vi "Main.vi"() -> ()   [LabVIEW 2020]
uses:
  Def/MHL_Data.ctl
  Def/Queue_Function Def.ctl
  Def/Queue_Method Def.ctl
  Def/Saving Type.ctl
  Def/Return(Watch Dog).ctl
  Def/Event Log.ctl
  Def/Error handler.ctl
  Objects/Saving Function/Saving OO/Save as csv/Save as csv.lvclass
  D:/Projects/practice/QMH+Producer_consumer/Multiple queues_PS/Objects/Saving Function/Saving OO/Saving OO.lvclass
  Def/Queue_Def.ctl
  <userlib>/_MGI/Timing/MGI Wait/MGI Wait (U32).vi
  Objects/Saving Function/Saving OO/Save as txt/Save as txt.lvclass
  Objects/Saving Function/Saving OO/Saving OO.lvclass
panel:
  in  "Connect/Reconnect":bool
  in  "Power":bool
  in  "Decrease Amplitude":bool
  in  "Add Amplitude":bool
  in  "Decrease Frequence":bool
  in  "Increase Frequence":bool
  out "Waveform":dynamicdata(graph)
  in  "MHL Data":T1={"Offset"=0.0, "Frequency"=10.1, "Amplitude"=1.0}
  out "Ver.#":string
  out "error out":errorcluster
  in  "error in (no error)":errorcluster
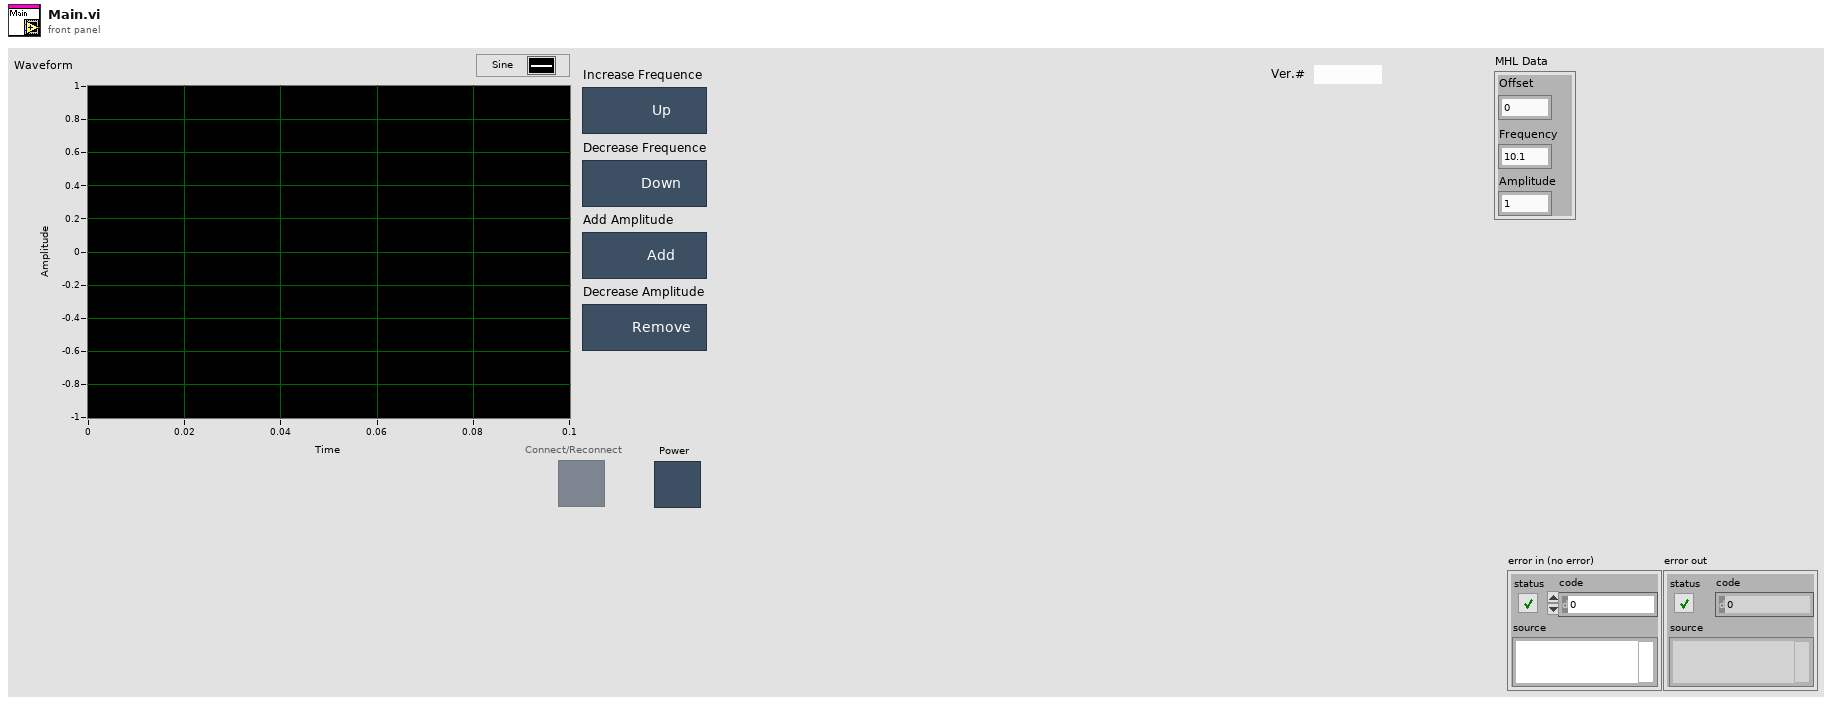
[diagram p1: front panel]
types:
  T1 = typedef "MHL_Data.ctl" = cluster{"Offset":dbl, "Frequency":dbl, "Amplitude":dbl}
  T2 = typedef "Error handler.ctl" = cluster{"code":i32, "source":string}
  T3 = typedef "Event Log.ctl" = cluster{"File paht":path}
  T4 = typedef "Queue_Method Def.ctl" = enum16{"Initialize", "Read", "Write", "Insert", "Get_Specific_Quene_Status", "Flush Speciffic Quene", "Release All Quenes"}
  T5 = typedef "Queue_Function Def.ctl" = enum16{"MHL", "Return(Watch dog)", "Event Log", "Error Log"}
  T6 = typedef "Return(Watch Dog).ctl" = cluster{string}
  T7 = typedef "Saving Type.ctl" = enum16{"Default", "txt", "csv"}
  T8 = typedef "Main_Data_Package.ctl" = cluster{"This Vi Ref Out":refnum<vi>, "Map Out":map{string, refnum<vi>}, "User Event Ref":refnum<user-event>, "User_Event Reg":refnum<event-registration>, "Event Log Path":path}
  T9 = enum8{"Enabled", "Disabled", "Disabled and Grayed Out"}
  T10 = typedef "Queue_Def.ctl" = cluster{"Message":string, "Data":variant}
  T11 = cluster{"Functions":T5, "Functions 2":T5, "Functions 3":T5, "Functions 4":T5}
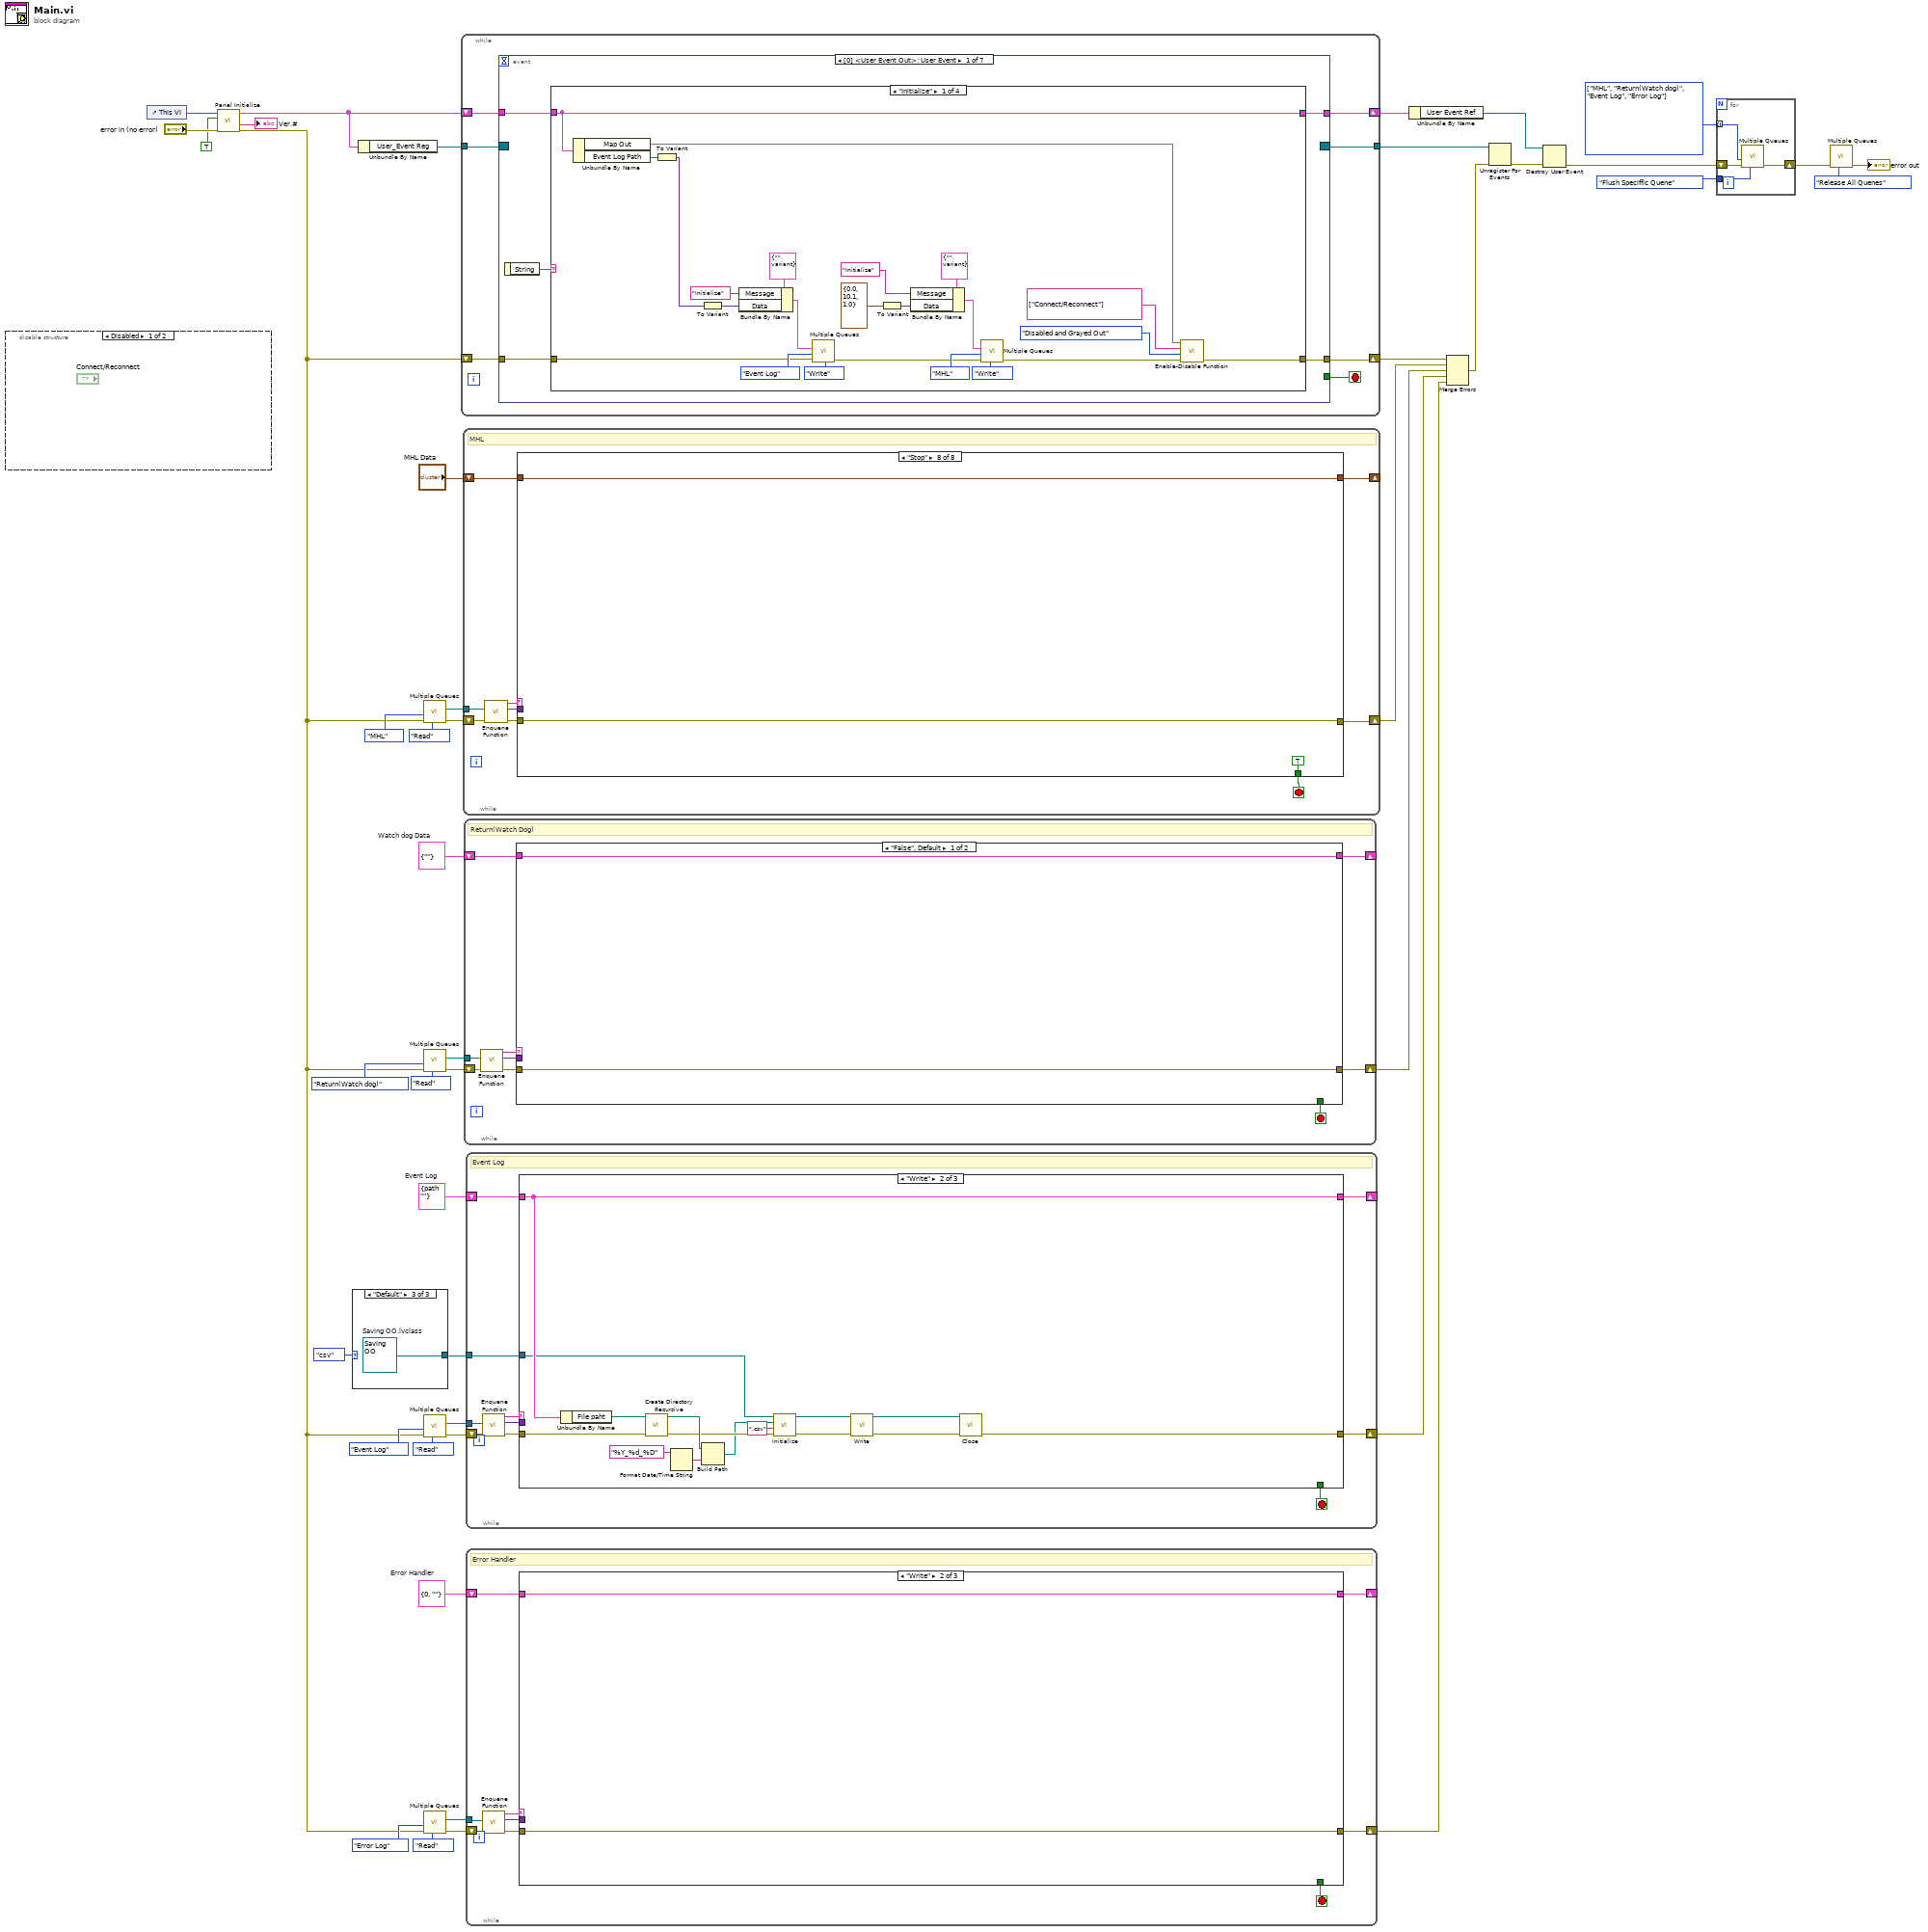
[diagram p0: block diagram]
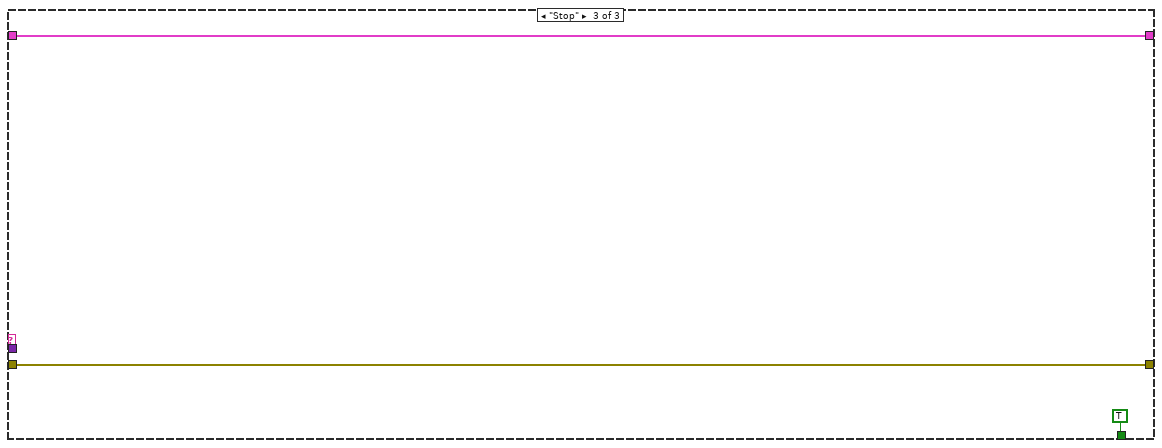
[diagram p3: hidden frame]
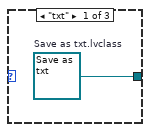
[diagram p5: hidden frame]
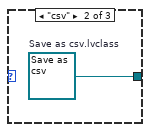
[diagram p6: hidden frame]
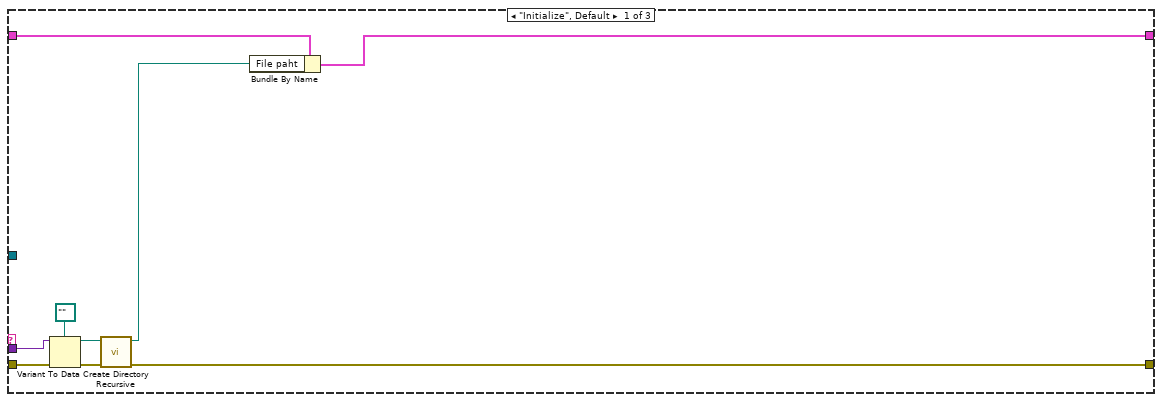
[diagram p7: hidden frame]
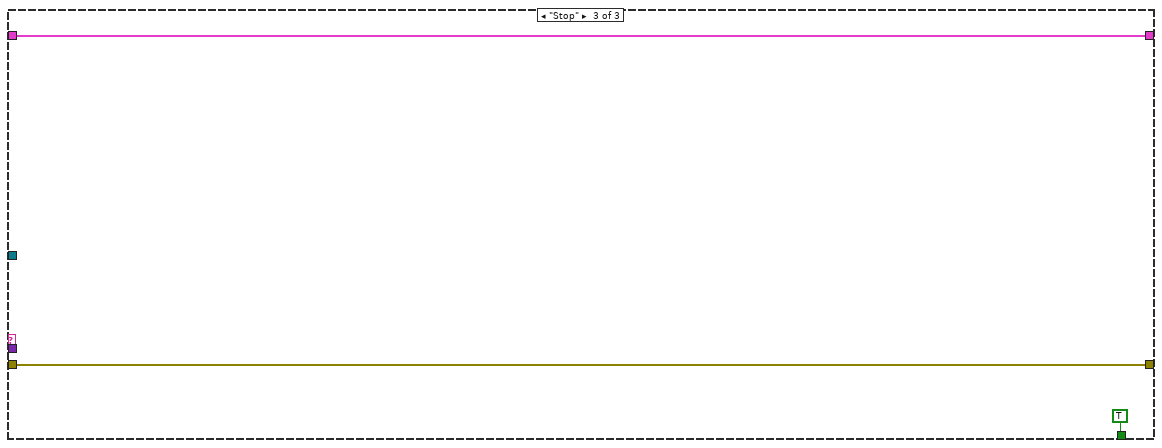
[diagram p8: hidden frame]
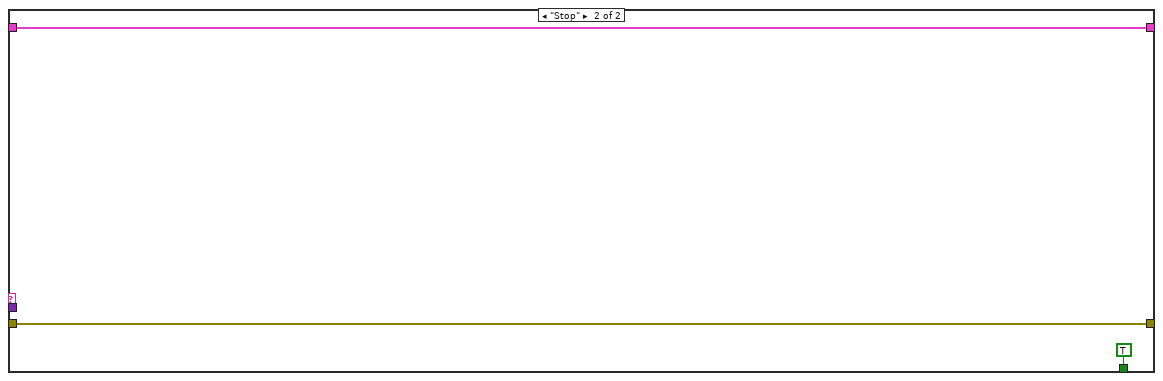
[diagram p9: hidden frame]
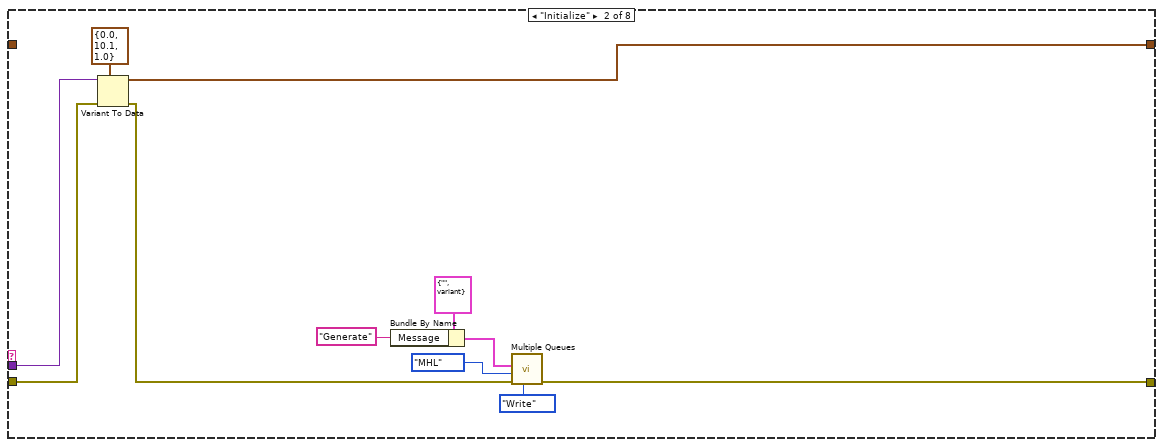
[diagram p11: hidden frame]
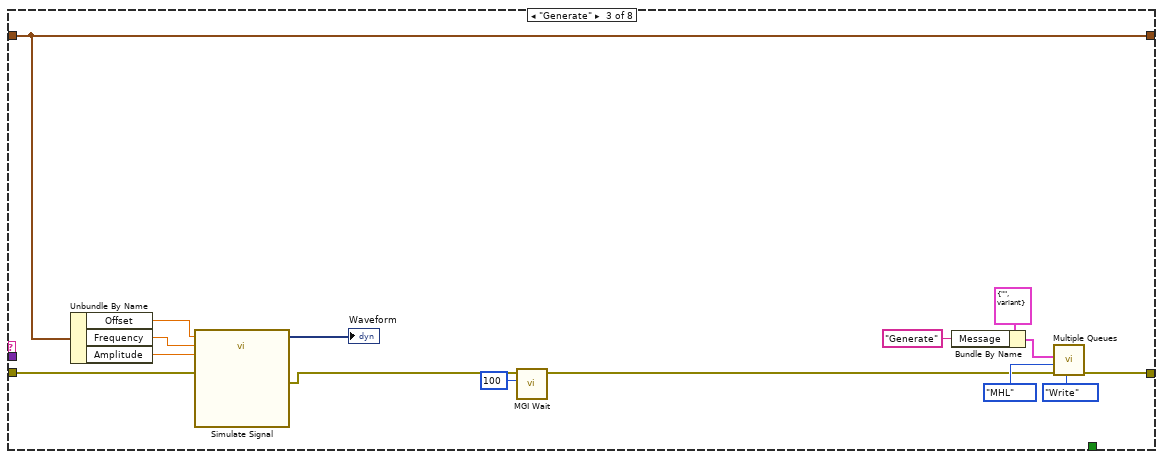
[diagram p12: hidden frame]
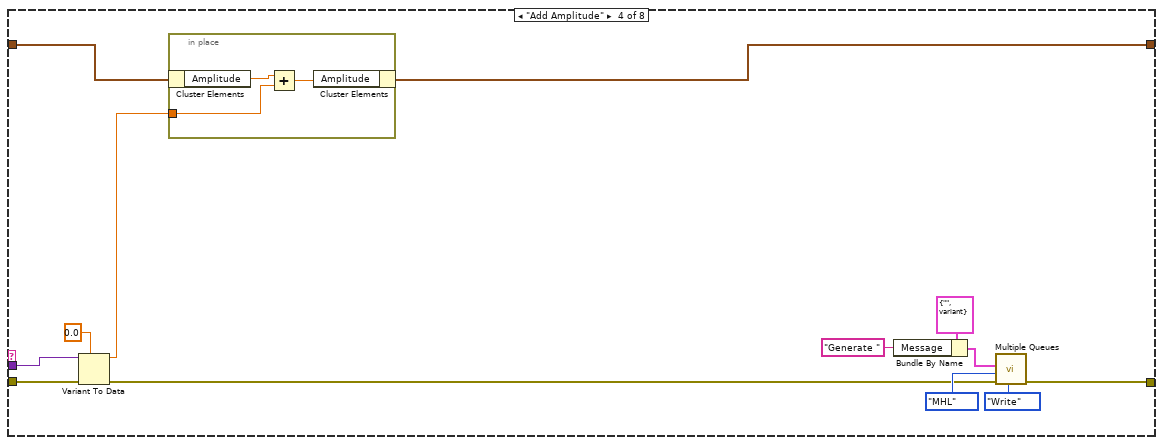
[diagram p13: hidden frame]
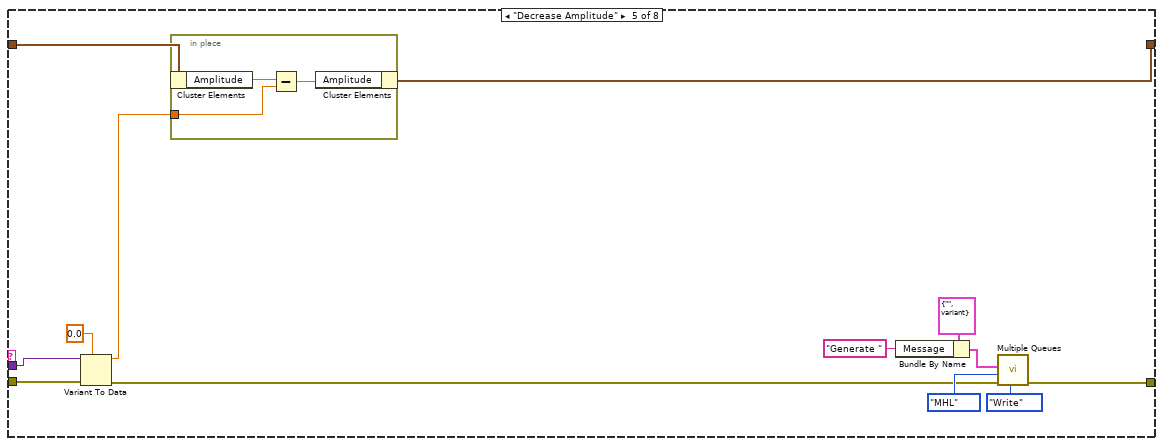
[diagram p14: hidden frame]
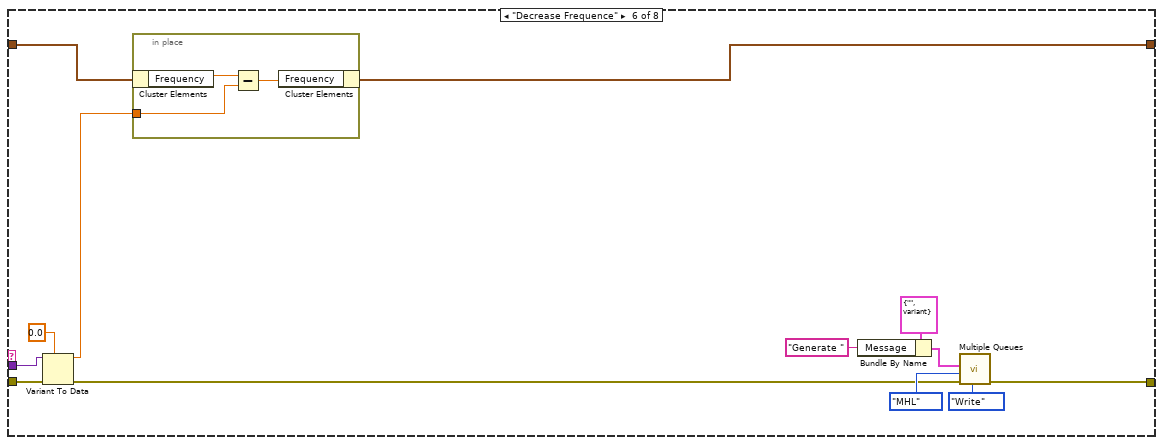
[diagram p15: hidden frame]
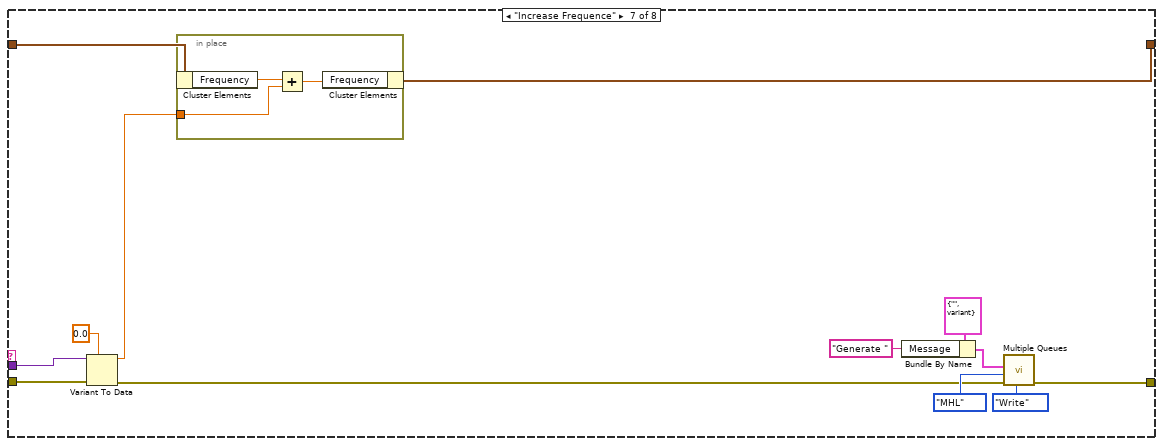
[diagram p16: hidden frame]
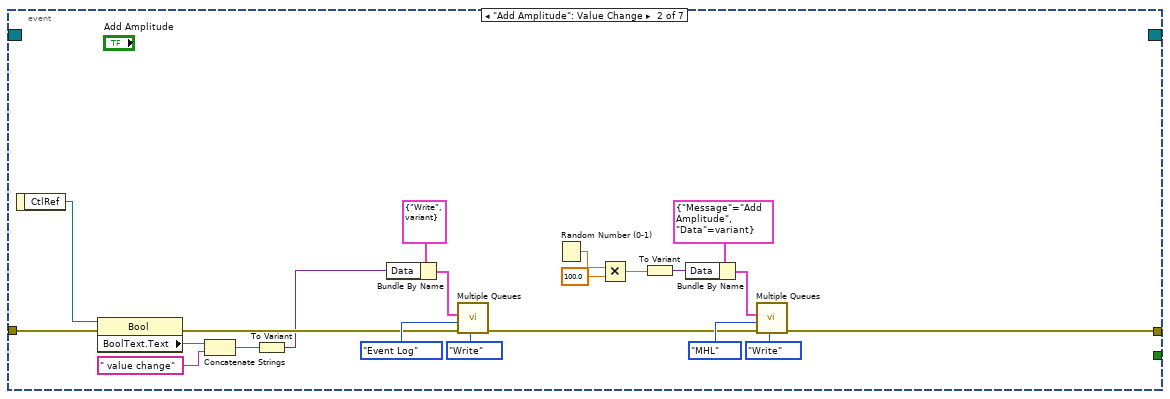
[diagram p20: hidden frame]
diagram:
  w1 = T2 {"code"=0, "source"=""}  # Error Handler
  w2 = T3 {"File paht"=path ""}  # Event Log
  w13 = T6 {""}  # Watch dog Data
  w38 = T5[] [enum."MHL", enum."Return(Watch dog)", enum."Event Log", enum."Error Log"] items=["MHL", "Return(Watch dog)", "Event Log", "Error Log"]
  n1 = disable-structure shown="Disabled" {
    frame Disabled {
    }
    frame Enabled {
    }
  }
  n2 = control-ref of="This VI"() -> (w45:refnum<vi>)
  n3 = call "Panel Initialize.vi"("error in"="error in (no error)", "Initialize All UI ?"=TRUE, "VI Ref"=w45) -> ("error out"=w5:errorcluster, "Ver.#"=→"Ver.#":string, "Structure Data"=w12:T8)  [unwired: 6 in]
  n4 = case shown="\"Default\"" Saving_Type."csv" ("Saving Type") {
    tunnel: [w46 w47 w48] -> w18
    frame "txt" {
      w46 = refnum<class "Save as txt.lvclass"> refnum  # Save as txt.lvclass
    }
    frame "csv" {
      w47 = refnum<class "Save as csv.lvclass"> refnum  # Save as csv.lvclass
    }
    frame "Default" {
      w48 = refnum<class "Saving OO.lvclass"> refnum  # Saving OO.lvclass
    }
  }
  n5 = Unbundle By Name(w12) -> ("User_Event Reg"=w9:refnum<event-registration>)
  n6 = call "Multiple Queues.vi"("Method"=Queue_Method_Def."Read", "error in"=w5, "Functions"=Queue_Function_Def."MHL") -> ("error out"=w14:errorcluster, "queue out"=w15:refnum<queue>)  [unwired: 6 in, 1 out]
  n7 = call "Multiple Queues.vi"("Method"=Queue_Method_Def."Read", "error in"=w5, "Functions"=Queue_Function_Def."Return(Watch dog)") -> ("error out"=w28:errorcluster, "queue out"=w27:refnum<queue>)  [unwired: 6 in, 1 out]
  n8 = call "Multiple Queues.vi"("Method"=Queue_Method_Def."Read", "error in"=w5, "Functions"=Queue_Function_Def."Event Log") -> ("error out"=w21:errorcluster, "queue out"=w22:refnum<queue>)  [unwired: 6 in, 1 out]
  n9 = call "Multiple Queues.vi"("Method"=Queue_Method_Def."Read", "error in"=w5, "Functions"=Queue_Function_Def."Error Log") -> ("error out"=w6:errorcluster, "queue out"=w3:refnum<queue>)  [unwired: 6 in, 1 out]
  n10 = while {
    tunnel: [w54] -> w42
    shift-right: [w52] -> w41
    shift-left: w5 -> [w53]
    shift-right: [w50] -> w11
    shift-left: w12 -> [w51]
    tunnel: w9 -> [w49]
    stop <- w55 stop-if-true
    n11 = event shown="[0] <User Event Out>: User Event" {
      selector: w49 -> [_ _ _ _ _ _ _]
      dyn-events: [_ _ _ _ _ _ _] -> w54
      timeout: _ -> [_ _ _ _ _ _ _]
      tunnel: [_ _ _ _ _ TRUE ("Discard?") w155] -> w55
      tunnel: w53 -> [w60 w95 w112 w122 w132 w145 w154]
      tunnel: [w59 w97 w111 w121 w131 w144 w153] -> w52
      tunnel: w51 -> [w57 _ _ _ _ _ _]
      tunnel: [w56 _ _ _ _ _ _] -> w50
      event User Event {
        n12 = event-data() -> ("String"=w58:string)  [unwired: 1 in]
        n13 = case shown="\"Initialize\"" w58 {
          tunnel: w60 -> [w71 w85 w87 w89]
          tunnel: [w66 w85 w87 w89] -> w59
          tunnel: [w65 w84 w86 w88] -> w56
          tunnel: w57 -> [w65 w84 w86 w88]
          frame "Initialize" {
            n14 = Unbundle By Name(w65) -> ("Map Out"=w63:map{string, refnum<vi>}, "Event Log Path"=w64:path)
            n15 = To Variant(anything=w64) -> (Variant=w68:variant)
            n16 = To Variant(anything=w68) -> (Variant=w69:variant)
            n17 = Bundle By Name(cluster=T10 {"Message"="", "Data"=variant} ("Quenes"), "Message"="Initialize", "Data"=w69) -> (w72:T10)
            n18 = call "Multiple Queues.vi"("Method"=Queue_Method_Def."Write", "error in"=w71, "Functions"=Queue_Function_Def."Event Log", "Quenes"=w72) -> ("error out"=w70:errorcluster)  [unwired: 5 in, 2 out]
            n19 = To Variant(anything=T1 {"Offset"=0.0, "Frequency"=10.1, "Amplitude"=1.0} ("MHL Data")) -> (Variant=w79:variant)
            n20 = Bundle By Name(cluster=T10 {"Message"="", "Data"=variant} ("Quenes"), "Message"="Initialize", "Data"=w79) -> (w77:T10)
            n21 = call "Multiple Queues.vi"("Method"=Queue_Method_Def."Write", "error in"=w70, "Functions"=Queue_Function_Def."MHL", "Quenes"=w77) -> ("error out"=w67:errorcluster)  [unwired: 5 in, 2 out]
            n22 = call "Enable-Disable Function.vi"("error in"=w67, "Disabled"=T9."Disabled and Grayed Out", "Labels"=string[] ["Connect/Reconnect"], "Map Out"=w63) -> ("error out"=w66:errorcluster)  [unwired: 7 in]
          }
          frame "Write a Log" {
          }
          frame "Refresh" {
          }
          frame Default {
          }
        }
      }
      event "Add Amplitude": Value Change {
        n23 = event-data() -> ("CtlRef"=w94:refnum<vi>)  [unwired: 1 in]
        n24 = property class="Bool"(reference=w94, error in=w95) -> (error out=w96:errorcluster, "BoolText.Text"=w93:string)  [unwired: 1 out]
        n25 = Concatenate Strings(w93, " value change") -> (w91:string)
        n26 = To Variant(anything=w91) -> (Variant=w90:variant)
        n27 = Bundle By Name(cluster=T10 {"Message"="Write", "Data"=variant} ("Quenes"), "Data"=w90) -> (w102:T10)
        n28 = call "Multiple Queues.vi"("Method"=Queue_Method_Def."Write", "error in"=w96, "Functions"=Queue_Function_Def."Event Log", "Quenes"=w102) -> ("error out"=w98:errorcluster)  [unwired: 5 in, 2 out]
        n29 = Random Number (0-1)() -> (number: 0 to 1=w107:dbl)
        n30 = Multiply(x=w107, y=100.0) -> (x*y=w105:dbl)
        n31 = To Variant(anything=w105) -> (Variant=w104:variant)
        n32 = Bundle By Name(cluster=T10 {"Message"="Add Amplitude", "Data"=variant} ("Quenes"), "Data"=w104) -> (w103:T10)
        n33 = call "Multiple Queues.vi"("Method"=Queue_Method_Def."Write", "error in"=w98, "Functions"=Queue_Function_Def."MHL", "Quenes"=w103) -> ("error out"=w97:errorcluster)  [unwired: 5 in, 2 out]
      }
      event "Decrease Amplitude": Value Change {
        n34 = event-data() -> ()  [unwired: 1 in, 1 out]
        n35 = Random Number (0-1)() -> (number: 0 to 1=w117:dbl)
        n36 = Multiply(x=w117, y=50.0) -> (x*y=w115:dbl)
        n37 = To Variant(anything=w115) -> (Variant=w114:variant)
        n38 = Bundle By Name(cluster=T10 {"Message"="Decrease Amplitude", "Data"=variant} ("Quenes"), "Data"=w114) -> (w113:T10)
        n39 = call "Multiple Queues.vi"("Method"=Queue_Method_Def."Write", "error in"=w112, "Functions"=Queue_Function_Def."MHL", "Quenes"=w113) -> ("error out"=w111:errorcluster)  [unwired: 5 in, 2 out]
      }
      event "Increase Frequence": Value Change {
        n40 = event-data() -> ()  [unwired: 1 in, 1 out]
        n41 = Random Number (0-1)() -> (number: 0 to 1=w127:dbl)
        n42 = Multiply(x=w127, y=30.0) -> (x*y=w125:dbl)
        n43 = To Variant(anything=w125) -> (Variant=w124:variant)
        n44 = Bundle By Name(cluster=T10 {"Message"="Increase Frequence", "Data"=variant} ("Quenes"), "Data"=w124) -> (w123:T10)
        n45 = call "Multiple Queues.vi"("Method"=Queue_Method_Def."Write", "error in"=w122, "Functions"=Queue_Function_Def."MHL", "Quenes"=w123) -> ("error out"=w121:errorcluster)  [unwired: 5 in, 2 out]
      }
      event "Decrease Frequence": Value Change {
        n46 = event-data() -> ()  [unwired: 1 in, 1 out]
        n47 = Random Number (0-1)() -> (number: 0 to 1=w137:dbl)
        n48 = Multiply(x=w137, y=15.0) -> (x*y=w135:dbl)
        n49 = To Variant(anything=w135) -> (Variant=w134:variant)
        n50 = Bundle By Name(cluster=T10 {"Message"="Decrease Frequence", "Data"=variant} ("Quenes"), "Data"=w134) -> (w133:T10)
        n51 = call "Multiple Queues.vi"("Method"=Queue_Method_Def."Write", "error in"=w132, "Functions"=Queue_Function_Def."MHL", "Quenes"=w133) -> ("error out"=w131:errorcluster)  [unwired: 5 in, 2 out]
      }
      event "Power": Value Change {
        n52 = event-data() -> ()  [unwired: 1 in, 1 out]
        n53 = Cluster To Array(cluster=T11 {"Functions"=enum."MHL", "Functions 2"=enum."Return(Watch dog)", "Functions 3"=enum."Event Log", "Functions 4"=enum."Error Log"}) -> (array=w141:T5[])
        n54 = for {
          tunnel: w141 -> [w147] mode=indexing
          tunnel: w145 -> [w150]
          tunnel: [w149] -> w144
          n55 = call "Multiple Queues.vi"("Method"=Queue_Method_Def."Insert", "error in"=w150, "Functions"=w147, "Quenes"=T10 {"Message"="Stop", "Data"=variant}) -> ("error out"=w149:errorcluster)  [unwired: 5 in, 2 out]
        }
      }
      event Panel Close? {
        w155 = TRUE ("Discard?")
        n56 = event-data() -> ()  [unwired: 1 in, 1 out]
        n57 = Cluster To Array(cluster=T11 {"Functions"=enum."MHL", "Functions 2"=enum."Return(Watch dog)", "Functions 3"=enum."Event Log", "Functions 4"=enum."Error Log"}) -> (array=w151:T5[])
        n58 = for {
          tunnel: w151 -> [w157] mode=indexing
          tunnel: w154 -> [w160]
          tunnel: [w159] -> w153
          n59 = call "Multiple Queues.vi"("Method"=Queue_Method_Def."Insert", "error in"=w160, "Functions"=w157, "Quenes"=T10 {"Message"="Stop", "Data"=variant}) -> ("error out"=w159:errorcluster)  [unwired: 5 in, 2 out]
        }
        n60 = event-data("Discard?"=w155) -> ()  [unwired: 1 in, 1 out]
      }
    }
  }
  n61 = while {
    shift-right: [w168] -> w40
    shift-left: w14 -> [w162]
    shift-right: [w164] -> _
    shift-left: "MHL Data" -> [w161]
    tunnel: w15 -> [w163]
    stop <- w169 stop-if-true
    # "MHL"
    n62 = call "Enquene Function.vi"("error in (no error)"=w162, "Queue"=w163) -> ("error out"=w167:errorcluster, "Data"=w165:variant, "Message"=w166:string)  [unwired: 7 in]
    n63 = case shown="\"Stop\"" w166 {
      tunnel: [_ _ _ _ _ _ _ TRUE] -> w169
      tunnel: [w171 w177 w193 w200 w216 w231 w246 w263] -> w168
      tunnel: w167 -> [w171 w179 w197 w210 w218 w233 w250 w263]
      tunnel: w165 -> [_ w181 _ w209 w217 w232 w249 _]
      tunnel: [w170 w178 w186 w198 w214 w230 w247 w262] -> w164
      tunnel: w161 -> [w170 _ w186 w199 w215 w234 w248 w262]
      frame Default {
      }
      frame "Initialize" {
        n64 = Variant To Data(error in=w179, type=T1 {"Offset"=0.0, "Frequency"=10.1, "Amplitude"=1.0} ("MHL Data"), Variant=w181) -> (data=w178:T1, error out=w180:errorcluster)
        n65 = Bundle By Name(cluster=T10 {"Message"="", "Data"=variant} ("Quenes"), "Message"="Generate") -> (w173:T10)
        n66 = call "Multiple Queues.vi"("Method"=Queue_Method_Def."Write", "error in"=w180, "Functions"=Queue_Function_Def."MHL", "Quenes"=w173) -> ("error out"=w177:errorcluster)  [unwired: 5 in, 2 out]
      }
      frame "Generate" {
        n67 = Unbundle By Name(w186) -> ("Offset"=w185:dbl, "Frequency"=w184:dbl, "Amplitude"=w183:dbl)
        n68 = call "Simulate Signal"("Offset"=w185, "Frequency"=w184, "Amplitude"=w183, "error in (no error)"=w197) -> ("Sine"=→"Waveform":dynamicdata, "error out"=w194:errorcluster)  [unwired: 10 in]
        n69 = call-poly <userlib>:"MGI Wait.vi"("ms"=u32 100, "Error In"=w194) -> ("Error Out"=w189:errorcluster)  [unwired: 5 in]
        n70 = Bundle By Name(cluster=T10 {"Message"="", "Data"=variant} ("Quenes"), "Message"="Generate") -> (w190:T10)
        n71 = call "Multiple Queues.vi"("Method"=Queue_Method_Def."Write", "error in"=w189, "Functions"=Queue_Function_Def."MHL", "Quenes"=w190) -> ("error out"=w193:errorcluster)  [unwired: 5 in, 2 out]
      }
      frame "Add Amplitude" {
        n72 = Variant To Data(error in=w210, type=0.0, Variant=w209) -> (data=w207:dbl, error out=w201:errorcluster)
        n73 = in-place {
          in-place-border: w207 -> [w213]
          n74 = in-place-cluster #1(w199) -> ("Amplitude"=w211:dbl)
          n75 = Add(x=w211, y=w213) -> (x+y=w212:dbl)
          n76 = in-place-cluster #1("Amplitude"=w212) -> (w198:T1)
        }
        n77 = Bundle By Name(cluster=T10 {"Message"="", "Data"=variant} ("Quenes"), "Message"="Generate ") -> (w202:T10)
        n78 = call "Multiple Queues.vi"("Method"=Queue_Method_Def."Write", "error in"=w201, "Functions"=Queue_Function_Def."MHL", "Quenes"=w202) -> ("error out"=w200:errorcluster)  [unwired: 5 in, 2 out]
      }
      frame "Decrease Amplitude" {
        n79 = Variant To Data(error in=w218, type=0.0, Variant=w217) -> (data=w225:dbl, error out=w219:errorcluster)
        n80 = in-place {
          in-place-border: w225 -> [w229]
          n81 = in-place-cluster #2(w215) -> ("Amplitude"=w227:dbl)
          n82 = Subtract(x=w227, y=w229) -> (x-y=w228:dbl)
          n83 = in-place-cluster #2("Amplitude"=w228) -> (w214:T1)
        }
        n84 = Bundle By Name(cluster=T10 {"Message"="", "Data"=variant} ("Quenes"), "Message"="Generate ") -> (w220:T10)
        n85 = call "Multiple Queues.vi"("Method"=Queue_Method_Def."Write", "error in"=w219, "Functions"=Queue_Function_Def."MHL", "Quenes"=w220) -> ("error out"=w216:errorcluster)  [unwired: 5 in, 2 out]
      }
      frame "Decrease Frequence" {
        n86 = Variant To Data(error in=w233, type=0.0, Variant=w232) -> (data=w241:dbl, error out=w235:errorcluster)
        n87 = in-place {
          in-place-border: w241 -> [w245]
          n88 = in-place-cluster #3(w234) -> ("Frequency"=w243:dbl)
          n89 = Subtract(x=w243, y=w245) -> (x-y=w244:dbl)
          n90 = in-place-cluster #3("Frequency"=w244) -> (w230:T1)
        }
        n91 = Bundle By Name(cluster=T10 {"Message"="", "Data"=variant} ("Quenes"), "Message"="Generate ") -> (w236:T10)
        n92 = call "Multiple Queues.vi"("Method"=Queue_Method_Def."Write", "error in"=w235, "Functions"=Queue_Function_Def."MHL", "Quenes"=w236) -> ("error out"=w231:errorcluster)  [unwired: 5 in, 2 out]
      }
      frame "Increase Frequence" {
        n93 = Variant To Data(error in=w250, type=0.0, Variant=w249) -> (data=w257:dbl, error out=w251:errorcluster)
        n94 = in-place {
          in-place-border: w257 -> [w261]
          n95 = in-place-cluster #4(w248) -> ("Frequency"=w259:dbl)
          n96 = Add(x=w259, y=w261) -> (x+y=w260:dbl)
          n97 = in-place-cluster #4("Frequency"=w260) -> (w247:T1)
        }
        n98 = Bundle By Name(cluster=T10 {"Message"="", "Data"=variant} ("Quenes"), "Message"="Generate ") -> (w252:T10)
        n99 = call "Multiple Queues.vi"("Method"=Queue_Method_Def."Write", "error in"=w251, "Functions"=Queue_Function_Def."MHL", "Quenes"=w252) -> ("error out"=w246:errorcluster)  [unwired: 5 in, 2 out]
      }
      frame "Stop" {
      }
    }
  }
  n100 = while {
    tunnel: w27 -> [w267]
    shift-right: [w271] -> w26
    shift-left: w28 -> [w273]
    shift-right: [w265] -> _
    shift-left: w13 -> [w266]
    stop <- w268 stop-if-true
    # "Return(Watch Dog)"
    n101 = call "Enquene Function.vi"("error in (no error)"=w273, "Queue"=w267) -> ("error out"=w272:errorcluster, "Data"=w269:variant, "Message"=w270:string)  [unwired: 7 in]
    n102 = case shown="\"False\", Default" w270 {
      tunnel: [w275 w278] -> w271
      tunnel: w272 -> [w275 w278]
      tunnel: w269 -> [_ _]
      tunnel: [_ TRUE] -> w268
      tunnel: w266 -> [w274 w276]
      tunnel: [w274 w276] -> w265
      frame "False", Default {
      }
      frame "Stop" {
      }
    }
  }
  n103 = while {
    shift-right: [w286] -> w20
    shift-left: w21 -> [w288]
    tunnel: w22 -> [w281]
    tunnel: w18 -> [w282]
    shift-right: [w279] -> _
    shift-left: w2 -> [w280]
    stop <- w283 stop-if-true
    # "Event Log"
    n104 = call "Enquene Function.vi"("error in (no error)"=w288, "Queue"=w281) -> ("error out"=w287:errorcluster, "Data"=w284:variant, "Message"=w285:string)  [unwired: 7 in]
    n105 = case shown="\"Write\"" w285 {
      tunnel: [w290 w303 w314] -> w286
      tunnel: w287 -> [w294 w305 w314]
      tunnel: w284 -> [w293 _ _]
      tunnel: [_ _ TRUE] -> w283
      tunnel: w282 -> [_ w299 _]
      tunnel: w280 -> [w291 w302 w313]
      tunnel: [w292 w302 w313] -> w279
      frame "Initialize", Default {
        n106 = Variant To Data(error in=w294, type=path "", Variant=w293) -> (data=w296:path, error out=w295:errorcluster)
        n107 = call <vilib>:"Create Directory Recursive.vi"("error in (no error)"=w295, "directory"=w296) -> ("error out"=w290:errorcluster, "directory copy"=w289:path)  [unwired: 3 in, 1 out]
        n108 = Bundle By Name(cluster=w291, "File paht"=w289) -> (w292:T3)
      }
      frame "Write" {
        n109 = Unbundle By Name(w302) -> ("File paht"=w300:path)
        n110 = call <vilib>:"Create Directory Recursive.vi"("error in (no error)"=w305, "directory"=w300) -> ("error out"=w304:errorcluster, "directory copy"=w310:path)  [unwired: 3 in, 1 out]
        n111 = Format Date/Time String(time format string (%c)="%Y_%d_%D") -> (date/time string=w311:string)  [unwired: 2 in]
        n112 = Build Path(base path=w310, name or relative path=w311) -> (appended path=w301:path)
        n113 = call-dynamic "Initialize.vi"("error in (no error)"=w304, "type"=".csv", "Path"=w301, "Saving OO in"=w299) -> ("error out"=w307:errorcluster, "Saving OO out"=w309:refnum<class "Saving OO.lvclass">)  [unwired: 6 in]
        n114 = call-dynamic "Write.vi"("error in (no error)"=w307, "Saving OO in"=w309) -> ("error out"=w306:errorcluster, "Saving OO out"=w308:refnum<class "Saving OO.lvclass">)  [unwired: 8 in]
        n115 = call-dynamic "Close.vi"("error in (no error)"=w306, "Saving OO in"=w308) -> ("error out"=w303:errorcluster)  [unwired: 8 in, 1 out]
      }
      frame "Stop" {
      }
    }
  }
  n116 = while {
    shift-right: [w322] -> w4
    shift-left: w6 -> [w324]
    tunnel: w3 -> [w318]
    shift-right: [w316] -> _
    shift-left: w1 -> [w317]
    stop <- w319 stop-if-true
    # "Error Handler"
    n117 = call "Enquene Function.vi"("error in (no error)"=w324, "Queue"=w318) -> ("error out"=w323:errorcluster, "Data"=w320:variant, "Message"=w321:string)  [unwired: 7 in]
    n118 = case shown="\"Write\"" w321 {
      tunnel: [w326 w328 w330] -> w322
      tunnel: w323 -> [w326 w328 w330]
      tunnel: w320 -> [_ _ _]
      tunnel: [_ _ TRUE] -> w319
      tunnel: w317 -> [w325 w327 w329]
      tunnel: [w325 w327 w329] -> w316
      frame "Initialize", Default {
      }
      frame "Write" {
      }
      frame "Stop" {
      }
    }
  }
  n119 = Unbundle By Name(w11) -> ("User Event Ref"=w10:refnum<user-event>)
  n120 = Merge Errors(w41, w40, w26, w20, w4) -> (w39:errorcluster)
  n121 = Unregister For Events(event registration refnum=w42, error in=w39) -> (error out=w43:errorcluster)
  n122 = Destroy User Event(user event=w10, error in=w43) -> (error out=w37:errorcluster)
  n123 = for {
    tunnel: w38 -> [w335] mode=indexing
    shift-right: [w333] -> w36
    shift-left: w37 -> [w334]
    tunnel: Queue_Method_Def."Flush Speciffic Quene" ("Method") -> [w332]
    n124 = call "Multiple Queues.vi"("Method"=w332, "error in"=w334, "Functions"=w335) -> ("error out"=w333:errorcluster)  [unwired: 6 in, 2 out]
  }
  n125 = call "Multiple Queues.vi"("Method"=Queue_Method_Def."Release All Quenes", "error in"=w36) -> ("error out"=→"error out":errorcluster)  [unwired: 7 in, 2 out]
